vi "to string.vi"(8 "error in":errorcluster, 11 "Standard Engine Repo Data in":refnum<class "synchronous engine configuration.lvclass">) -> (0 "error out":errorcluster, 1 "data":string, 2 "version":string, 3 "Standard Engine Repo Data out":refnum<class "synchronous engine configuration.lvclass">)   [LabVIEW 2014, in "synchronous engine configuration.lvclass"]
uses:
  synchronous engine configuration.lvclass
  synchronous engine configuration.lvclass/synchronous engine configuration.ctl
  Engine Configuration/engine configuration.lvclass
  <vilib>/NI/Configuration Framework/serializable configuration/NISE_CEF_serializable configuration.lvclass
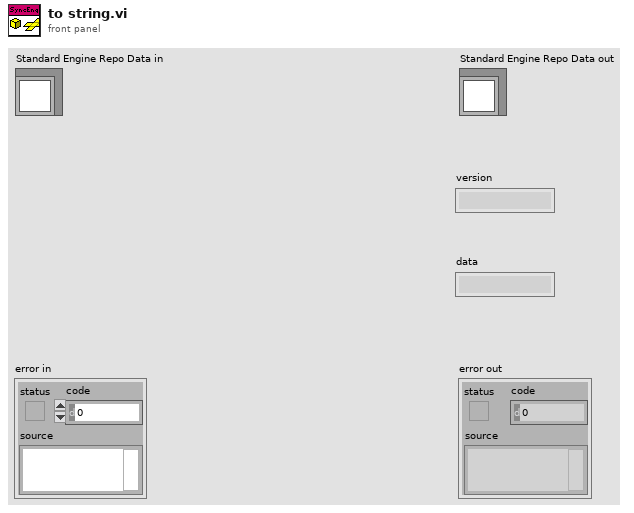
[diagram p1: front panel]
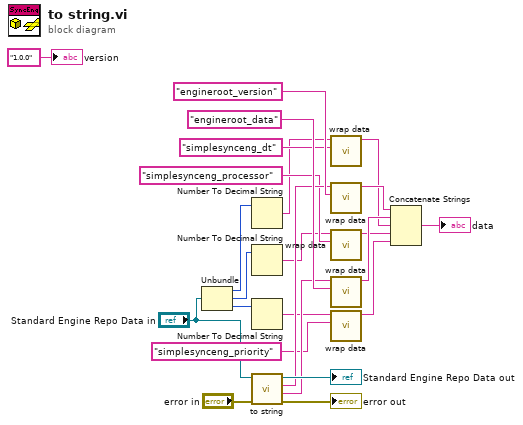
[diagram p0: block diagram]
diagram:
  n1 = Unbundle("Standard Engine Repo Data in") -> (w3:u32, w2:i32, w1:i32)
  n2 = Number To Decimal String(number=w3) -> (decimal integer string=w8:string)  [unwired: 1 in]
  n3 = Number To Decimal String(number=w2) -> (decimal integer string=w9:string)  [unwired: 1 in]
  n4 = Number To Decimal String(number=w1) -> (decimal integer string=w10:string)  [unwired: 1 in]
  n5 = call-parent "to string.vi"("error in"="error in", "engine configuration in"="Standard Engine Repo Data in") -> ("error out"=→"error out":errorcluster, "data"=w16:string, "version"=w17:string, "engine configuration out"=→"Standard Engine Repo Data out":refnum<class "synchronous engine configuration.lvclass">)  [unwired: 6 in]
  n6 = call <vilib>:"wrap data.vi"("identifier"="simplesynceng_dt" ("additional identifier"), "data to wrap"=w8) -> ("wrapped data"=w7:string)  [unwired: 9 in]
  n7 = call <vilib>:"wrap data.vi"("identifier"="engineroot_version" ("additional identifier"), "data to wrap"=w17) -> ("wrapped data"=w18:string)  [unwired: 9 in]
  n8 = call <vilib>:"wrap data.vi"("identifier"="simplesynceng_processor" ("additional identifier"), "data to wrap"=w9) -> ("wrapped data"=w6:string)  [unwired: 9 in]
  n9 = call <vilib>:"wrap data.vi"("identifier"="engineroot_data" ("additional identifier"), "data to wrap"=w16) -> ("wrapped data"=w19:string)  [unwired: 9 in]
  n10 = call <vilib>:"wrap data.vi"("identifier"="simplesynceng_priority" ("additional identifier"), "data to wrap"=w10) -> ("wrapped data"=w5:string)  [unwired: 9 in]
  n11 = Concatenate Strings(w18, w19, w7, w6, w5) -> (→"data":string)
  "version" <- "1.0.0" ("version")
